vi "Add status to name.vi"(10 "Status":T1, 11 "Name":string) -> (3 "Name with status":string)   [LabVIEW 2013, in "PL Framework Configuration Tool.lvlib"]
uses:
  PL Framework Configuration Tool.lvlib
  Glyphs Status.ctl
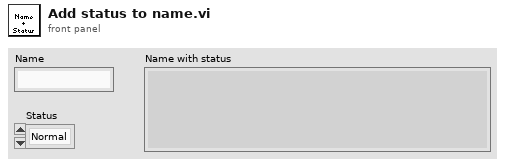
[diagram p1: front panel]
types:
  T1 = typedef "PL Framework Configuration Tool.lvlib/Glyphs Status.ctl" = enum16{"Normal", "Error"}
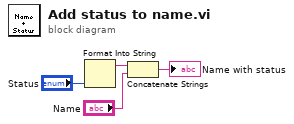
[diagram p0: block diagram]
diagram:
  n1 = Format Into String("Status") -> (resulting string=w3:string)  [unwired: 3 in, 1 out]
  n2 = Concatenate Strings(w3, "Name") -> (→"Name with status":string)
